vi "PWM Start.vi"(8 "error in (no error)":errorcluster, 9 "RunTimeUs":u32, 10 "ChannelMask":u8, 11 "DevHandle":i32) -> (0 "error out":errorcluster, 3 "function return":i32)   [LabVIEW 2010, in "usb2pwm.lvlib"]
doc: "int WINAPI PWM_Start(int DevHandle,unsigned char ChannelMask,unsigned int RunTimeUs);"
uses:
  usb2pwm.lvlib
  libs/msvc_x86/USB2XXX.dll
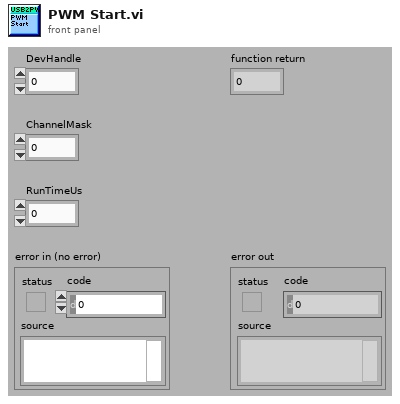
[diagram p1: front panel]
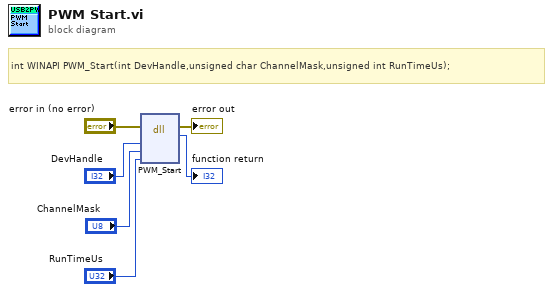
[diagram p0: block diagram]
diagram:
  # "int WINAPI PWM_Start(int DevHandle,unsigned char ChannelMask,unsigned int RunTimeUs);"
  n1 = dll-call lib="E:/OtherWork/STM32/USB2XXX_Example/sdk/libs/msvc_x86/USB2XXX.*" fn="PWM_Start"(error in="error in (no error)", "DevHandle"="DevHandle", "ChannelMask"="ChannelMask", "RunTimeUs"="RunTimeUs") -> (error out=→"error out":errorcluster, →"function return":i32)  [unwired: 5 in, 1 out]
